vi "InitConstants.vi"   [LabVIEW 2019]
uses:
  constants.vi
  sensors.vi
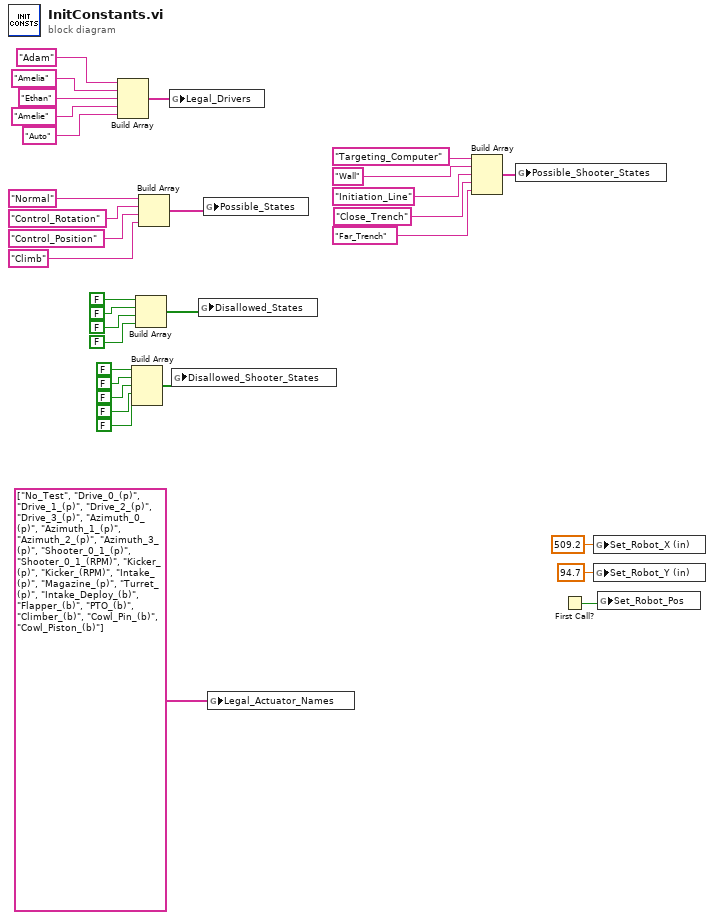
[diagram p0: block diagram]
diagram:
  n1 = Build Array("Adam" ("element"), "Amelia" ("element"), "Ethan", "Amelie" ("element"), "Auto" ("element")) -> (w30:string[])
  n2 = Build Array(FALSE, FALSE, FALSE, FALSE ("element"), FALSE ("element")) -> (w20:bool[])
  n3 = Build Array(FALSE, FALSE, FALSE, FALSE ("element")) -> (w25:bool[])
  n4 = Build Array("Normal", "Control_Rotation", "Control_Position", "Climb") -> (w26:string[])
  n5 = global write "constants.vi" "Legal_Drivers"(w30) -> ()
  n6 = global write "constants.vi" "Disallowed_Shooter_States"(w20) -> ()
  n7 = global write "constants.vi" "Disallowed_States"(w25) -> ()
  n8 = global write "constants.vi" "Possible_States"(w26) -> ()
  n9 = global write "constants.vi" "Legal_Actuator_Names"(string[] ["No_Test", "Drive_0_(p)", "Drive_1_(p)", "Drive_2_(p)", "Drive_3_(p)", "Azimuth_0_(p)", "Azimuth_1_(p)", "Azimuth_2_(p)", "Azimuth_3_(p)", "Shooter_0_1_(p)", "Shooter_0_1_(RPM)", "Kicker_(p)", "Kicker_(RPM)", "Intake_(p)", "Magazine_(p)", "Turret_(p)", "Intake_Deploy_(b)", "Flapper_(b)", "PTO_(b)", "Climber_(b)", "Cowl_Pin_(b)", "Cowl_Piston_(b)"] ("appended array")) -> ()
  n10 = Build Array("Targeting_Computer", "Wall", "Initiation_Line", "Close_Trench" ("element"), "Far_Trench" ("element")) -> (w12:string[])
  n11 = global write "constants.vi" "Possible_Shooter_States"(w12) -> ()
  n12 = First Call?() -> (First Call?: T/F=w3:bool)
  n13 = global write "sensors.vi" "Set_Robot_X (in)"(509.2 ("Set_Robot_X (in)")) -> ()
  n14 = global write "sensors.vi" "Set_Robot_Y (in)"(94.7 ("Set_Robot_Y (in)")) -> ()
  n15 = global write "sensors.vi" "Set_Robot_Pos"(w3) -> ()
